vi "Load_Analogue_Data_2_Time_traces.vi"(1 "Voltage Array":dbl[][](array[numeric]), 2 "Sampling Rate (Hz)":dbl[](array[numeric])) -> ()   [LabVIEW 2017]
uses:
  Globals/Meas_global.vi
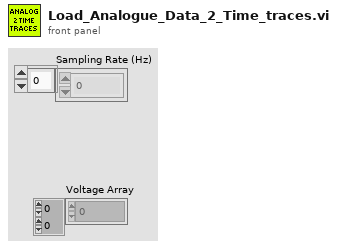
[diagram p1: front panel]
types:
  T1 = typedef "Analysis_info_cluster.ctl" = cluster{"Colour":u32, "Inst type":T2, "Inst name":string, "Symbol":string, "Code name":string, "Extra Info":string, "Inst Array":T3, "Extra Titles":string[], "Extra Values":string[], "U":dbl, "u^2":dbl, "u^3":dbl, "u^4":dbl, "Skew_u":dbl, "Kurt_u":dbl, "Sd Error in Mean":dbl, "% u'/U":dbl, "X":dbl, "Y":dbl, "Z":dbl, "Timescale integral Estimate":dbl, "Sd Error in Variance":dbl, "Calib File":path, "Calib Constants":dbl[], "Output Position":bool, "Full Stats":bool, "Av Sampling Rate":dbl, "Av No of Samples":dbl, "Total Meas Time (s)":dbl, "ADAM Ch Name":string, "Max value":dbl, "Min value":dbl, "Req Sample Rate Hz":dbl, "Sync Delay Time (s)":dbl, "Ch No":i16, "Device ID":string, "Use Latest Calib":bool, "Port":string}
  T2 = typedef "Inst_type.ctl" = enum16{"Propeller anemometer", "Raw voltage", "Pressure Transducer", "Pitot-static tube", "Preston tube", "Hot wire", "Cross wire 1", "Cross wire 2", "Generic Linear", "Generic Polynomial", "Generic BackPoly", "Fast FID", "Thermocouple", "Cold wire", "Pulsed Wire", "LDA Vel", "LDA Tran time", "LDA Arr time", "Microphone"}
  T3 = typedef "Instrument_Array.ctl" = enum16{"PWA", "LDA", "Analogue"}
  T4 = typedef "Time_Trace_Cluster.ctl" = cluster{"Weighting":dbl[], "Time (s)":dbl[], "Voltage":dbl[], "Eng Values":dbl[]}
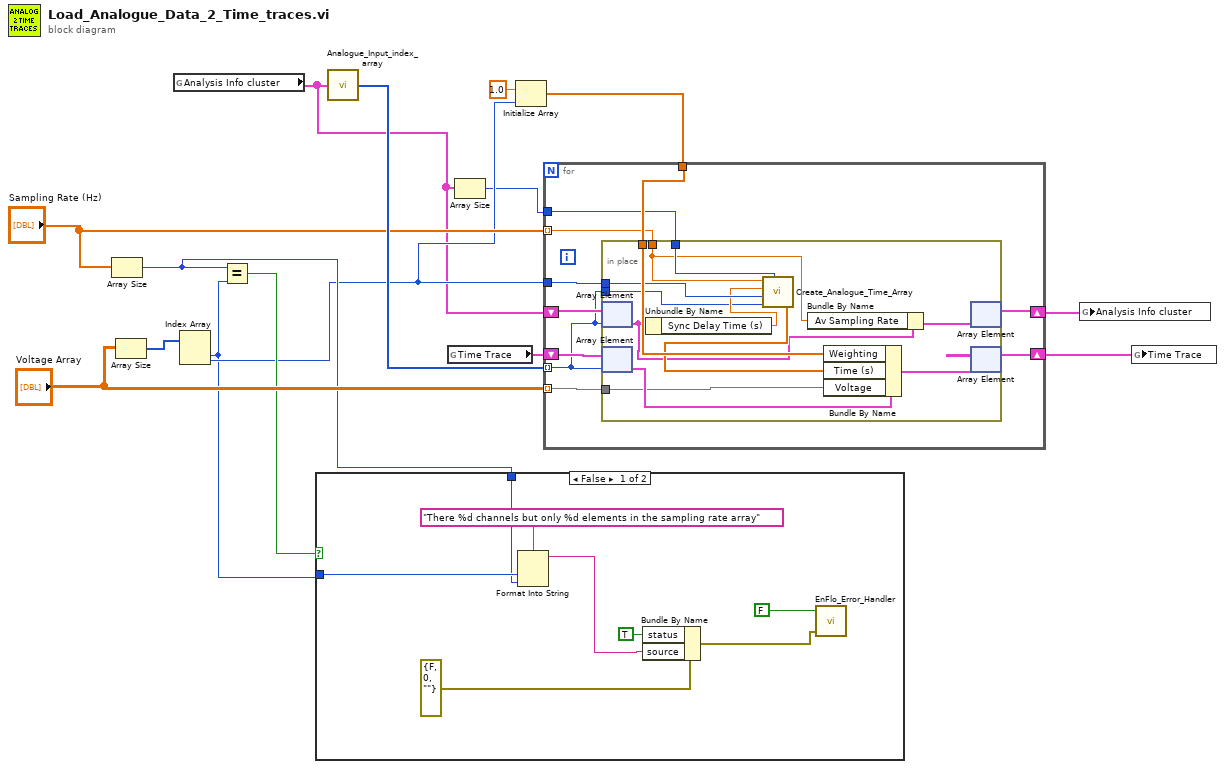
[diagram p0: block diagram]
diagram:
  n1 = Array Size(array="Sampling Rate (Hz)") -> (size(s)=w6:i32)
  n2 = Array Size(array="Voltage Array") -> (size(s)=w9:i32[])
  n3 = global read "Meas_global.vi" "Analysis Info cluster"() -> (w2:T1[])
  n4 = Index Array(array=w9) -> (element #1=w4:i32, element #2=w5:i32)  [unwired: 2 in]
  n5 = Equal?(x=w6, y=w4) -> (x = y?=w7:bool)
  n6 = case shown="False" w7 {
    tunnel: w4 -> [w20 _]
    tunnel: w6 -> [w19 _]
    frame False {
      n7 = Format Into String(format string="There %d channels but only %d elements in the sampling rate array", w20, w19) -> (resulting string=w17:string)  [unwired: 2 in, 1 out]
      n8 = Bundle By Name(cluster=errorcluster {"status"=FALSE, "code"=0, "source"=""} ("error in (no error)"), "status"=TRUE, "source"=w17) -> (w16:errorcluster)
      n9 = call "EnFlo_Error_Handler.vi"("error in (no error)"=w16, "Dialog Box (T)"=FALSE) -> ()  [unwired: 1 in, 3 out]
    }
    frame True {
    }
  }
  n10 = call "Analogue_Input_index_array.vi"("Analysis Info cluster"=w2) -> ("Array"=w10:i32[])
  n11 = global read "Meas_global.vi" "Time Trace"() -> (w12:T4[])
  n12 = Array Size(array=w2) -> (size(s)=w1:i32)
  n13 = Initialize Array(1.0 ("element"), w5) -> (w15:dbl[])
  n14 = for {
    shift-right: [w31] -> w13
    shift-left: w12 -> [w33]
    tunnel: w10 -> [w24] mode=indexing
    tunnel: "Voltage Array" -> [w32] mode=indexing
    tunnel: w15 -> [w30]
    tunnel: "Sampling Rate (Hz)" -> [w29] mode=indexing
    tunnel: w5 -> [w28]
    tunnel: w1 -> [w27]
    shift-right: [w25] -> w3
    shift-left: w2 -> [w26]
    n15 = in-place {
      in-place-border: w32 -> [w44]
      in-place-border: w30 -> [w42]
      in-place-border: w29 -> [w35]
      in-place-border: w28 -> [w41]
      in-place-border: w27 -> [w40]
      in-place-border: w24 -> [w34]
      n16 = in-place-array #1(w26, w24) -> (w37:T1)
      n17 = in-place-array #2(w33, w24) -> (w45:T4)
      n18 = Unbundle By Name(w37) -> ("Sync Delay Time (s)"=w38:dbl)
      n19 = call "Create_Analogue_Time_Array.vi"("Sampling Rate (Hz)"=w35, "Sync Delay (s)"=w38, "No of Samples"=w41, "Index"=w34, "Total No of Chs"=w40) -> ("Times"=w39:dbl[])
      n20 = Bundle By Name(cluster=w37, "Av Sampling Rate"=w35) -> (w36:T1)
      n21 = Bundle By Name(cluster=w45, "Weighting"=w42, "Time (s)"=w39, "Voltage"=w44) -> (w43:T4)
      n22 = in-place-array #1(w36) -> (w25:T1[])  [unwired: 1 out]
      n23 = in-place-array #2(w43) -> (w31:T4[])  [unwired: 1 out]
    }
  }
  n24 = global write "Meas_global.vi" "Analysis Info cluster"(w3) -> ()
  n25 = global write "Meas_global.vi" "Time Trace"(w13) -> ()
